vi "Init.vi"(6 "Template Path":path, 8 "Project:Active Project":refnum<vi>, 9 "NI.LV.Dialog Instance":refnum<vi>, 10 "Template Name":string) -> (3 "Script out":refnum<class "Script.lvclass">)   [LabVIEW 2021, in "_Template.lvlib" / "Script.lvlib" / "Script.lvclass"]
uses:
  Script.lvclass
  Script.lvclass/Script.ctl
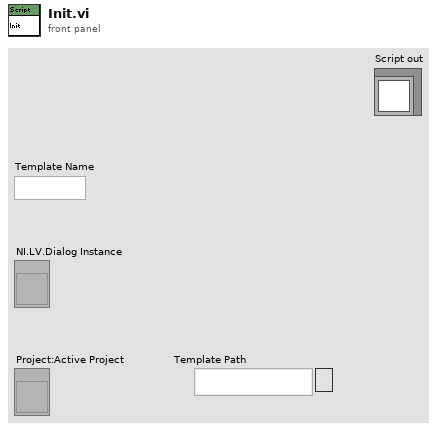
[diagram p1: front panel]
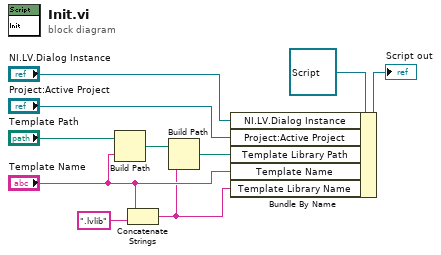
[diagram p0: block diagram]
diagram:
  n1 = Build Path(base path="Template Path", name or relative path="Template Name") -> (appended path=w8:path)
  n2 = Concatenate Strings("Template Name", ".lvlib" ("string")) -> (w3:string)
  n3 = Build Path(base path=w8, name or relative path=w3) -> (appended path=w6:path)
  n4 = Bundle By Name(cluster=refnum<class "Script.lvclass"> refnum ("_Create From Template.lvlib:Script Strategy.lvlib:First Library Script Strategy.lvclass"), "NI.LV.Dialog Instance"="NI.LV.Dialog Instance", "Project:Active Project"="Project:Active Project", "Template Library Path"=w6, "Template Name"="Template Name", "Template Library Name"=w3) -> (→"Script out":refnum<class "Script.lvclass">)
